vi "CalculoRampaSubida.vi"(10 "TempoRampa":dbl, 11 "PicoMax":dbl) -> (3 "XY Graph":cluster{"X":dbl, "Y":dbl}[](graph))   [LabVIEW 2019]
panel:
  in  "Array":cluster{"X":dbl, "Y":dbl}[](array[cluster])
  # "segundos"
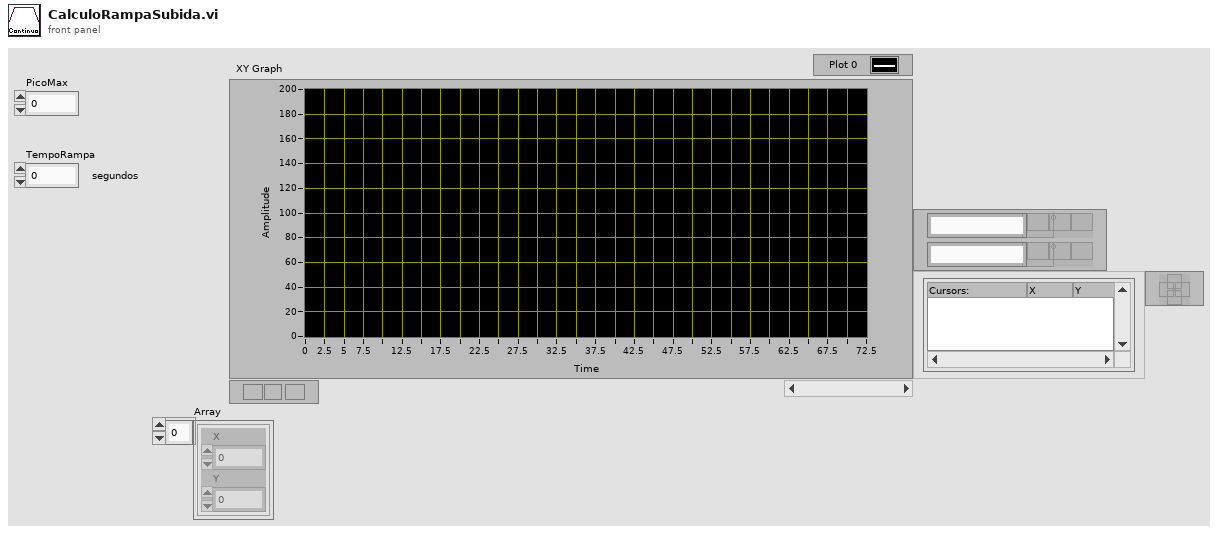
[diagram p1: front panel]
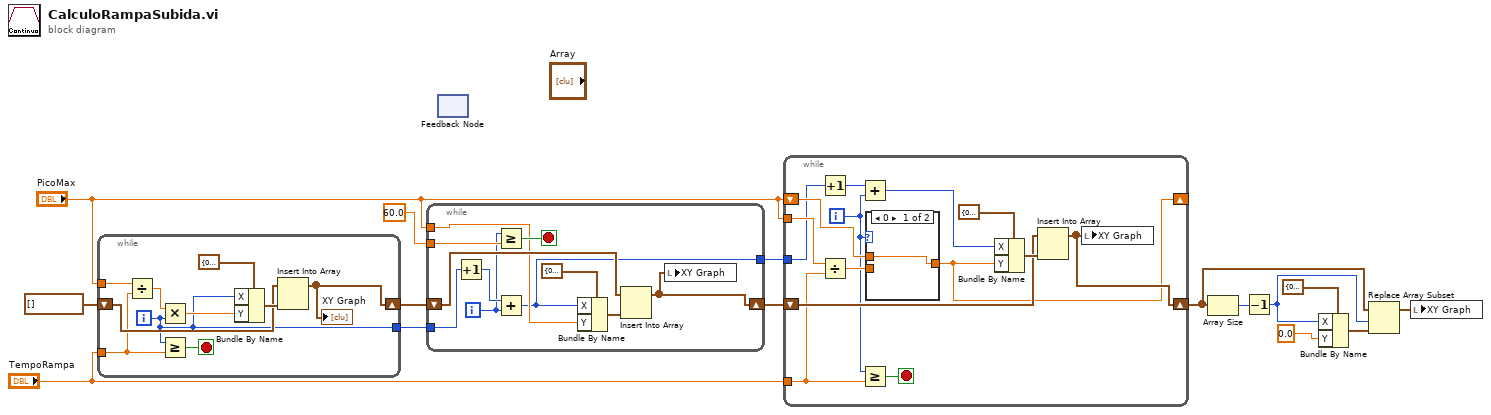
[diagram p0: block diagram]
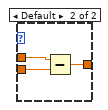
[diagram p2: hidden frame]
diagram:
  n1 = while {
    tunnel: "PicoMax" -> [w19]
    tunnel: "TempoRampa" -> [w18]
    shift-right: [w22] -> w13
    shift-left: cluster{"X":dbl, "Y":dbl}[] [] -> [w21]
    tunnel: [w16] -> w8
    i -> [w16]
    stop <- w25 stop-if-true
    n2 = Divide(x=w19, y=w18) -> (x/y=w17:dbl)
    n3 = Multiply(x=w17, y=w16) -> (x*y=w20:dbl)
    n4 = Greater Or Equal?(x=w16, y=w18) -> (x >= y?=w25:bool)
    n5 = Bundle By Name(cluster=cluster{"X":dbl, "Y":dbl} {"X"=0.0, "Y"=0.0} ("new element/subarray"), "X"=w16, "Y"=w20) -> (w23:cluster{"X":dbl, "Y":dbl})
    n6 = Insert Into Array(array=w21, new element=w23) -> (w22:cluster{"X":dbl, "Y":dbl}[])  [unwired: 1 in]
    "XY Graph" <- w22
  }
  n7 = while {
    tunnel: 60.0 ("Numeric 2") -> [w32]
    shift-right: [w30] -> w10
    shift-left: w13 -> [w33]
    tunnel: "PicoMax" -> [w31]
    tunnel: w8 -> [w29]
    tunnel: [w26] -> w7
    i -> [w27]
    stop <- w36 stop-if-true
    n8 = Increment(x=w29) -> (x+1=w28:i32)
    n9 = Greater Or Equal?(x=w27, y=w32) -> (x >= y?=w36:bool)
    n10 = Add(x=w28, y=w27) -> (x+y=w26:i32)
    n11 = Bundle By Name(cluster=cluster{"X":dbl, "Y":dbl} {"X"=0.0, "Y"=0.0} ("new element/subarray"), "X"=w26, "Y"=w31) -> (w34:cluster{"X":dbl, "Y":dbl})
    n12 = Insert Into Array(array=w33, new element=w34) -> (w30:cluster{"X":dbl, "Y":dbl}[])  [unwired: 1 in]
    n13 = local write "XY Graph"(w30) -> ()
  }
  n14 = feedback-in #1() -> ()  [unwired: 1 out]
  n15 = feedback #1() -> ()  [unwired: 2 in]
  n16 = while {
    tunnel: "TempoRampa" -> [w45]
    shift-right: [w46] -> w9
    shift-left: w10 -> [w47]
    tunnel: "PicoMax" -> [w44]
    shift-right: [w41] -> _
    shift-left: "PicoMax" -> [w42]
    tunnel: w7 -> [w40]
    i -> [w37]
    stop <- w50 stop-if-true
    n17 = Increment(x=w40) -> (x+1=w39:i32)
    n18 = Divide(x=w44, y=w45) -> (x/y=w43:dbl)
    n19 = Add(x=w39, y=w37) -> (x+y=w38:i32)
    n20 = Greater Or Equal?(x=w37, y=w45) -> (x >= y?=w50:bool)
    n21 = case shown="0" w37 {
      tunnel: w43 -> [_ w54]
      tunnel: w42 -> [w51 w53]
      tunnel: [w51 w52] -> w41
      frame 0 {
      }
      frame Default {
        n22 = Subtract(x=w53, y=w54) -> (x-y=w52:dbl)
      }
    }
    n23 = Bundle By Name(cluster=cluster{"X":dbl, "Y":dbl} {"X"=0.0, "Y"=0.0} ("new element/subarray"), "X"=w38, "Y"=w41) -> (w48:cluster{"X":dbl, "Y":dbl})
    n24 = Insert Into Array(array=w47, new element=w48) -> (w46:cluster{"X":dbl, "Y":dbl}[])  [unwired: 1 in]
    n25 = local write "XY Graph"(w46) -> ()
  }
  n26 = Array Size(array=w9) -> (size(s)=w6:i32)
  n27 = Decrement(x=w6) -> (x-1=w1:i32)
  n28 = Bundle By Name(cluster=cluster{"X":dbl, "Y":dbl} {"X"=0.0, "Y"=0.0} ("new element/subarray"), "X"=w1, "Y"=0.0) -> (w3:cluster{"X":dbl, "Y":dbl})
  n29 = Replace Array Subset(array=w9, new element=w3, index=w1) -> (w2:cluster{"X":dbl, "Y":dbl}[])
  n30 = local write "XY Graph"(w2) -> ()
